vi "set_value.vi"() -> ()   [LabVIEW 2019]
panel:
  in  "stop":bool
  out "spill_id":i32
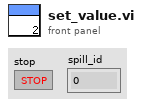
[diagram p1: front panel]
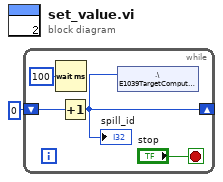
[diagram p0: block diagram]
diagram:
  n1 = while {
    shift-right: [w4] -> _
    shift-left: 0 -> [w3]
    stop <- "stop" stop-if-true
    n2 = Wait (ms)(milliseconds to wait=u32 100) -> ()  [unwired: 1 out]
    n3 = Increment(x=w3) -> (x+1=w4:i32)
    "spill_id" <- w4
    n4 = shared-variable ".\\E1039TargetComputerShared.lvlib\\spill_id"(w4) -> ()  [unwired: 1 in, 1 out]
  }
